vi "Preprocess_and_Convert_IMAQ_Image_to_Array.vi"(7 "PreProcessing_Options":T2 {"Dataset_Stats"."stds"."R" format="%#_3g"; "Dataset_Stats"."stds"."G" format="%#_3g"; "Dataset_Stats"."stds"."B" format="%#_3g"; "Dataset_Stats"."means"."R" format="%#_3g"; "Dataset_Stats"."means"."G" format="%#_3g"; "Dataset_Stats"."means"."B" format="%#_3g"; "Interpolation Type" items=["Zero Order", "Bi-Linear", "Quadratic", "Cubic Spline"]}, 8 "error in (no error)":errorcluster, 11 "Imaq Image In":T1) -> (0 "error out":errorcluster, 2 "Norm_Img_Out":sgl[][][](array[numeric]), 3 "Imaq Image Out":T1, 5 "dT_Preprocessing":dbl)   [LabVIEW 2020]
uses:
  <vilib>/Ngene/DeepLTK Anomaly Detection Addon/DeepLTK_Anomaly_Detection_Addon/API/Controls/NNPC_PreProcessing_Options.ctl
  <vilib>/Ngene/Deep Learning Toolkit/Toolkit/NN_Data/API/NN_Dims(C,H,W).ctl
  <vilib>/Ngene/DeepLTK Anomaly Detection Addon/DeepLTK_Anomaly_Detection_Addon/API/Controls/NNPC_DS_Stats.ctl
  <vilib>/Ngene/DeepLTK Anomaly Detection Addon/DeepLTK_Anomaly_Detection_Addon/API/Controls/Image_Stats_RGB.ctl
  <vilib>/vision/Image Controls.llb/IMAQ Image.ctl
  <vilib>/vision/NI_Vision_Development_Module.lvlib
  <vilib>/Ngene/Deep Learning Toolkit/Toolkit/Deep_Learning_Toolkit_by_Ngene.lvlib
  <vilib>/Ngene/DeepLTK Anomaly Detection Addon/DeepLTK_Anomaly_Detection_Addon/DeepLTK_Anomaly_Detection_Addon.lvlib
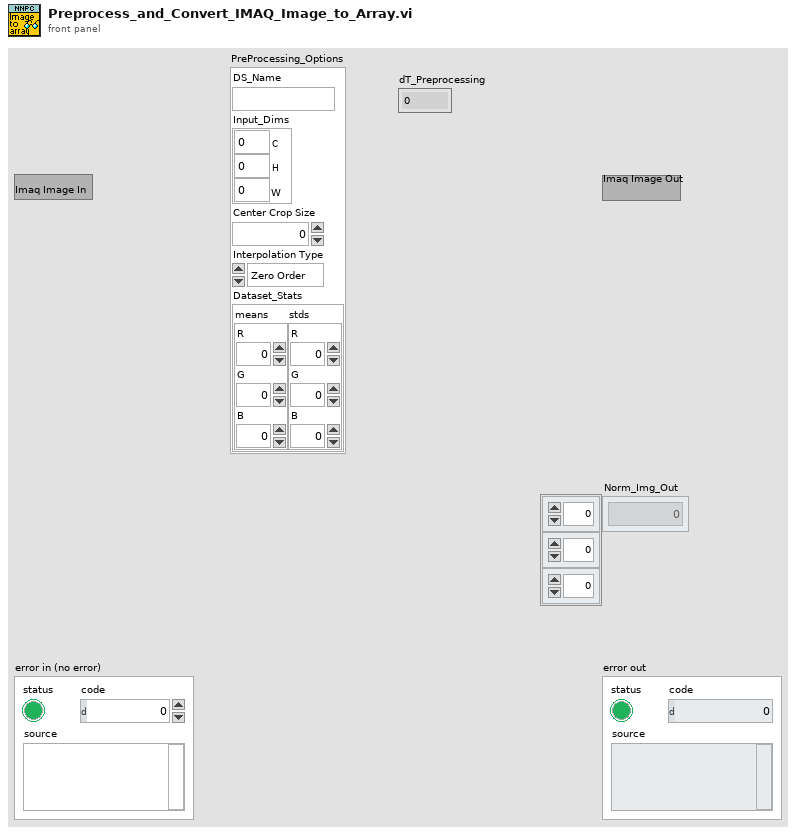
[diagram p1: front panel]
types:
  T1 = typedef "IMAQ Image.ctl" = refnum<image>
  T2 = typedef "DeepLTK_Anomaly_Detection_Addon.lvlib/NNPC_PreProcessing_Options.ctl" = cluster{"DS_Name":string, "Input_Dims":T3, "Center Crop Size":i32, "Interpolation Type":u32, "Dataset_Stats":T4}
  T3 = typedef "Deep_Learning_Toolkit_by_Ngene.lvlib/NN_Dims(C,H,W).ctl" = cluster{"C":i32, "H":i32, "W":i32}
  T4 = typedef "DeepLTK_Anomaly_Detection_Addon.lvlib/NNPC_DS_Stats.ctl" = cluster{"means":T5, "stds":T5}
  T5 = typedef "DeepLTK_Anomaly_Detection_Addon.lvlib/Image_Stats_RGB.ctl" = cluster{"R":sgl, "G":sgl, "B":sgl}
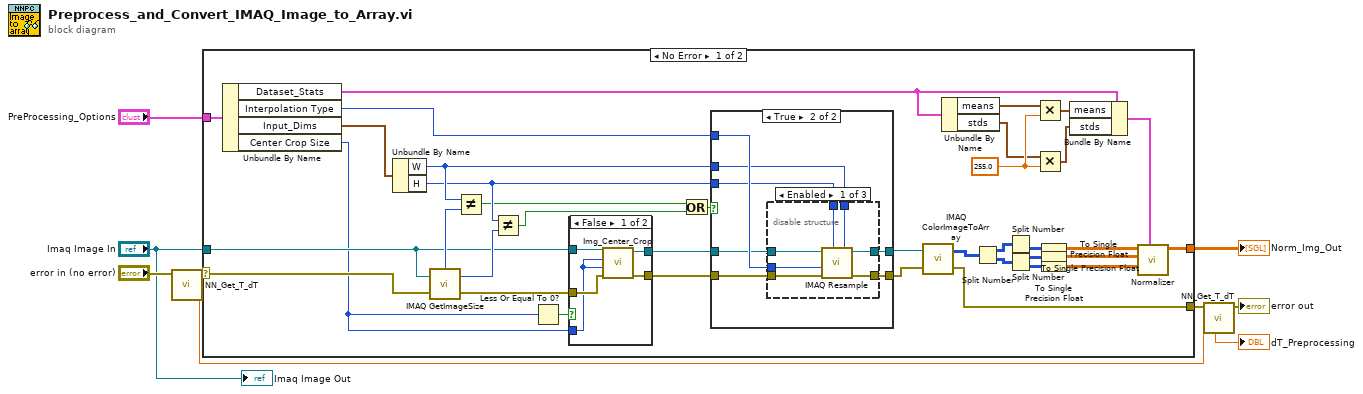
[diagram p0: block diagram]
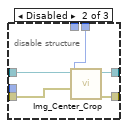
[diagram p4: hidden frame]
diagram:
  n1 = call <vilib>:"NN_Get_T_dT.vi"("error in (no error)"="error in (no error)") -> ("T_out"=w2:dbl, "error out"=w3:errorcluster)  [unwired: 6 in, 1 out]
  n2 = case shown="No Error" w3 {
    selector: w3 -> [w16 w77]
    tunnel: "PreProcessing_Options" -> [w46 _]
    tunnel: "Imaq Image In" -> [w15 _]
    tunnel: [w23 w77] -> w8
    tunnel: [w22 _] -> w7
    frame No Error {
      w38 = sgl 255.0 ("R")
      n3 = Unbundle By Name(w46) -> ("Dataset_Stats"=w39:T4, "Interpolation Type"=w28:u32, "Input_Dims"=w29:T3, "Center Crop Size"=w10:i32)
      n4 = Unbundle By Name(w29) -> ("W"=w26:i32, "H"=w25:i32)
      n5 = call "IMAQ GetImageSize"("Image"=w15, "error in (no error)"=w16) -> ("Y Resolution"=w18:i32, "X Resolution"=w17:i32, "error out"=w13:errorcluster)  [unwired: 2 in]
      n6 = Not Equal?(x=w26, y=w17) -> (x != y?=w20:bool)
      n7 = Not Equal?(x=w25, y=w18) -> (x != y?=w19:bool)
      n8 = Less Or Equal To 0?(x=w10) -> (x <= 0?=w11:bool)
      n9 = case shown="False" w11 {
        tunnel: w15 -> [w51 w53]
        tunnel: [w50 w53] -> w14
        tunnel: w13 -> [w49 w52]
        tunnel: [w48 w52] -> w12
        tunnel: w10 -> [w47 _]
        frame False {
          n10 = call "Img_Center_Crop.vi"("error in (no error)"=w49, "y"=w47, "x"=w47, "Image In"=w51) -> ("error out"=w48:errorcluster, "Image Out"=w50:T1)  [unwired: 6 in]
        }
        frame True {
        }
      }
      n11 = Or(x=w20, y=w19) -> (x .or. y?=w21:bool)
      n12 = case shown="True" w21 {
        tunnel: w26 -> [_ w58]
        tunnel: w25 -> [_ w57]
        tunnel: [w54 w61] -> w24
        tunnel: [w55 w62] -> w27
        tunnel: w12 -> [w55 w56]
        tunnel: w14 -> [w54 w59]
        tunnel: w28 -> [_ w60]
        frame False {
        }
        frame True {
          n13 = disable-structure shown="Enabled" {
            disable-tunnel: w57 -> [w69 _ _]
            disable-tunnel: [w68 w74 w75] -> w62
            disable-tunnel: [w67 w73 w76] -> w61
            disable-tunnel: w56 -> [w66 w72 w75]
            disable-tunnel: w59 -> [w65 w71 w76]
            disable-tunnel: w60 -> [w64 _ _]
            disable-tunnel: w58 -> [w63 w70 _]
            frame Enabled {
              n14 = call "IMAQ Resample"("X Resolution"=w63, "Y Resolution"=w69, "error in (no error)"=w66, "Interpolation Type"=w64, "Image Src"=w65) -> ("error out"=w68:errorcluster, "Image Dst Out"=w67:T1)  [unwired: 5 in]
            }
            frame Disabled {
              n15 = call "Img_Center_Crop.vi"("y"=w72, "x"=w70, "Image In"=w71) -> ("error out"=w74:errorcluster, "Image Out"=w73:T1)  [unwired: 7 in]
            }
            frame Disabled {
            }
          }
        }
      }
      n16 = call "IMAQ ColorImageToArray"("Image"=w24, "error in (no error)"=w27) -> ("Image Pixels (U32)"=w35:u32[][], "error out"=w23:errorcluster)  [unwired: 2 in, 1 out]
      n17 = Unbundle By Name(w39) -> ("means"=w36:T5, "stds"=w37:T5)
      n18 = Split Number(x=w35) -> (hi(x)=w31:u16[][], lo(x)=w30:u16[][])
      n19 = Split Number(x=w31) -> (lo(x)=w32:u8[][])  [unwired: 1 out]
      n20 = Split Number(x=w30) -> (hi(x)=w33:u8[][], lo(x)=w34:u8[][])
      n21 = Multiply(x=w36, y=w38) -> (x*y=w41:T5)
      n22 = Multiply(x=w37, y=w38) -> (x*y=w42:T5)
      n23 = To Single Precision Float(number=w32) -> (single precision float=w43:sgl[][])
      n24 = To Single Precision Float(number=w33) -> (single precision float=w44:sgl[][])
      n25 = To Single Precision Float(number=w34) -> (single precision float=w45:sgl[][])
      n26 = Bundle By Name(cluster=w39, "means"=w41, "stds"=w42) -> (w40:T4)
      n27 = call "Normalizer.vi"("Dataset_Stats"=w40, "B"=w45, "G"=w44, "R"=w43) -> ("Norm_Img_Out"=w22:sgl[][][])  [unwired: 7 in]
    }
    frame Error {
    }
  }
  "Norm_Img_Out" <- w7
  n28 = call <vilib>:"NN_Get_T_dT.vi"("T_in"=w2, "error in (no error)"=w8) -> ("error out"=→"error out":errorcluster, "dT"=→"dT_Preprocessing":dbl)  [unwired: 5 in, 1 out]
  "Imaq Image Out" <- "Imaq Image In"
